vi "IsLogDigitalIOTriggered.vi"(9 "Digital IO Edge":T1, 10 "Digital IO Line":i32, 11 "Log Data":T2[](array[typedef])) -> (3 "Triggered?":bool)   [LabVIEW 2012]
uses:
  HardwareLogData.ctl
  HardwareDisplayData.ctl
  LogDigitalIOTriggerEdge.ctl
  LogLastPortGlobalAction.ctl
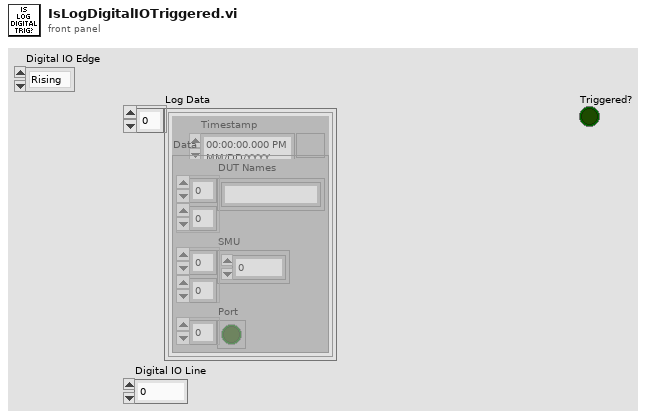
[diagram p1: front panel]
types:
  T1 = typedef "LogDigitalIOTriggerEdge.ctl" = enum16{"Rising", "Falling"}
  T2 = typedef "HardwareLogData.ctl" = cluster{"Timestamp":timestamp, "Data":T3}
  T3 = typedef "HardwareDisplayData.ctl" = cluster{"DUT Names":string[][], "SMU":dbl[][], "Port":bool[]}
  T4 = typedef "LogLastPortGlobalAction.ctl" = enum16{"Set", "Get"}
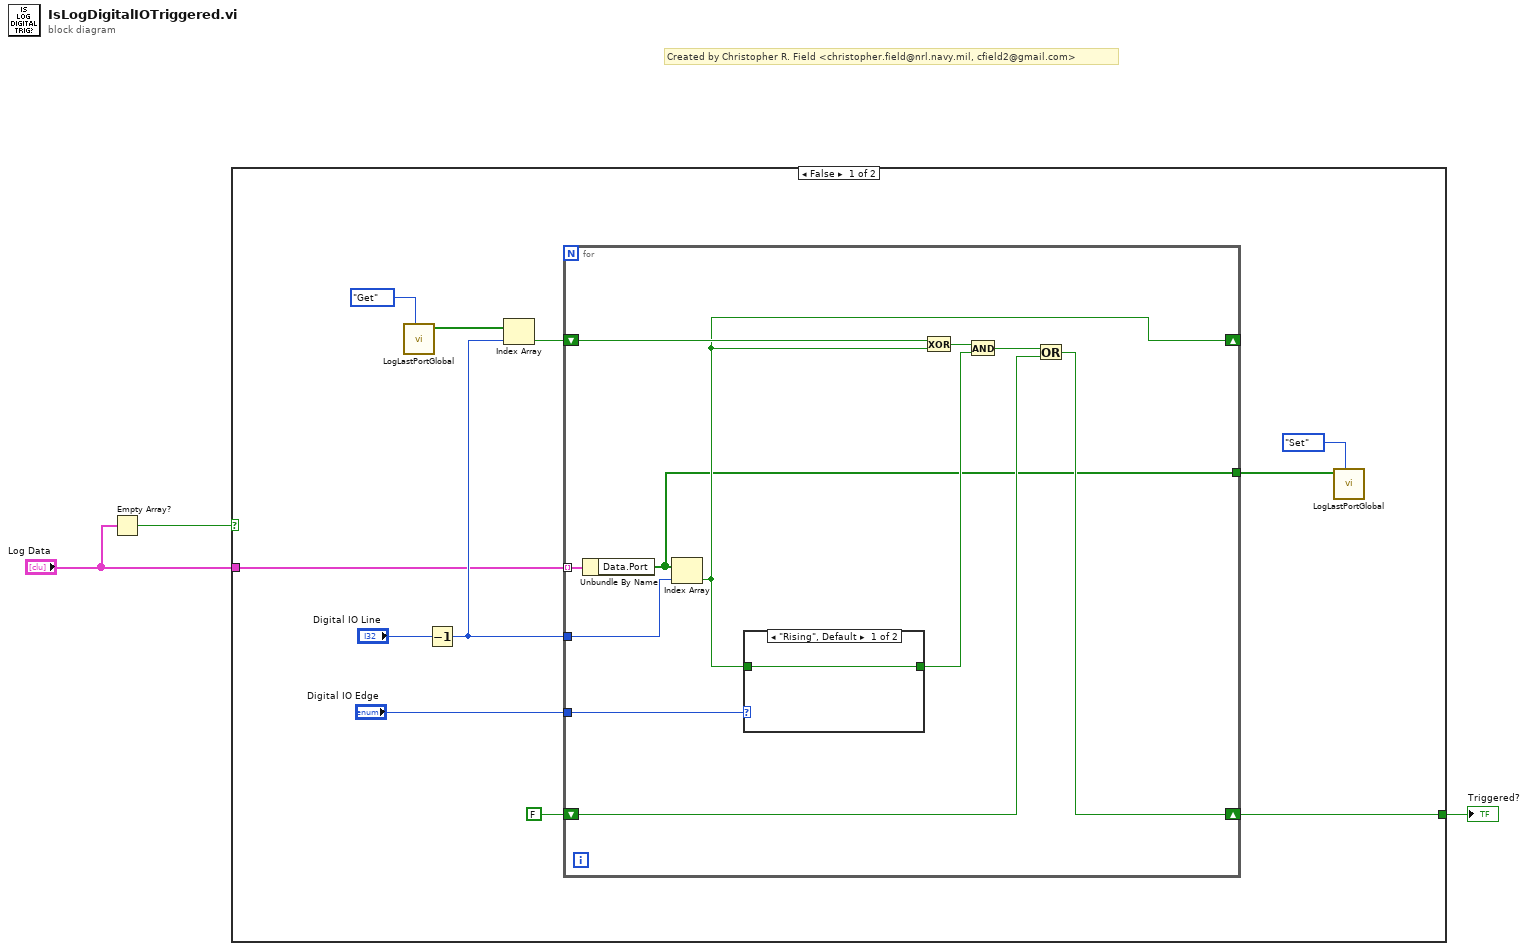
[diagram p0: block diagram]
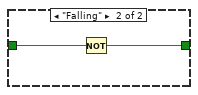
[diagram p2: hidden frame]
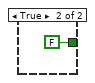
[diagram p3: hidden frame]
diagram:
  # "Created by Christopher R. Field <christopher.field@nrl.navy.mil, cfield2@gmail.com>"
  n1 = Empty Array?(array="Log Data") -> (empty?=w1:bool)
  n2 = case shown="False" w1 {
    tunnel: "Log Data" -> [w5 _]
    tunnel: [w4 FALSE] -> w3
    frame False {
      n3 = call "LogLastPortGlobal.vi"("Action"=LogLastPortGlobalAction."Get") -> ("Value Out"=w12:bool[])  [unwired: 10 in]
      n4 = Decrement(x="Digital IO Line") -> (x-1=w11:i32)
      n5 = Index Array(array=w12, index=w11) -> (element=w10:bool)
      n6 = for {
        tunnel: w5 -> [w25] mode=indexing
        tunnel: w11 -> [w24]
        shift-right: [w19] -> _
        shift-left: w10 -> [w23]
        tunnel: "Digital IO Edge" -> [w20]
        shift-right: [w16] -> w4
        shift-left: FALSE -> [w17]
        tunnel: [w15] -> w7
        n7 = Unbundle By Name(w25) -> ("Data.Port"=w15:bool[])
        n8 = Index Array(array=w15, index=w24) -> (element=w19:bool)
        n9 = case shown="\"Rising\", Default" w20 {
          tunnel: [w26 w28] -> w21
          tunnel: w19 -> [w26 w27]
          frame "Rising", Default {
          }
          frame "Falling" {
            n10 = Not(x=w27) -> (.not. x?=w28:bool)
          }
        }
        n11 = Exclusive Or(1:w19, 2:w23) -> (0:w22:bool)
        n12 = And(x=w22, y=w21) -> (x .and. y?=w18:bool)
        n13 = Or(x=w18, y=w17) -> (x .or. y?=w16:bool)
      }
      n14 = call "LogLastPortGlobal.vi"("Action"=LogLastPortGlobalAction."Set", "Set Value"=w7) -> ()  [unwired: 9 in, 1 out]
    }
    frame True {
    }
  }
  "Triggered?" <- w3
